vi "chart series set trendline intercept.vi"(8 "error in (no error)":errorcluster, 10 "intercept":dbl, 11 "series":u32) -> (0 "error out":errorcluster)   [LabVIEW 8.6]
doc: "void chart_series_set_trendline_intercept(lxw_chart_series series, double intercept);"
uses:
  pending_lvxlsxwriter/xlsxwriter.dll
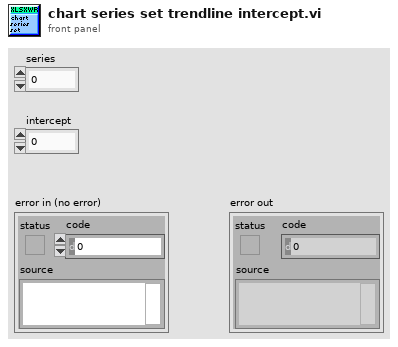
[diagram p1: front panel]
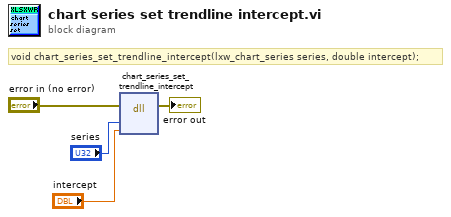
[diagram p0: block diagram]
diagram:
  # "void chart_series_set_trendline_intercept(lxw_chart_series series, double intercept);"
  n1 = dll-call lib="C:/Users/WDAGUtilityAccount/Desktop/pending_lvxlsxwriter/xlsxwriter.*" fn="chart_series_set_trendline_intercept"(error in="error in (no error)", "series"="series", "intercept"="intercept") -> (error out=→"error out":errorcluster)  [unwired: 5 in, 1 out]
